vi "Fanfare Sound Test.vi"   [LabVIEW 2014]
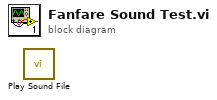
[diagram p0: block diagram]
diagram:
  n1 = call <vilib>:"Play Sound File.vi"() -> ()  [unwired: 10 in, 2 out]
